vi "Append Changed Item.vi"(6 "change type":T1, 7 "item name":string, 9 "new value":string, 10 "old value":string, 11 "refresh items in":T2[](array[typedef])) -> (2 "modify parent":bool, 3 "refresh items out":T2[](array[typedef]))   [LabVIEW 2020, in "AIM MIL-STD-1553 System Explorer.lvlib" / "Implementation.lvlib" / "Refresh.lvlib"]
uses:
  Refresh.lvlib
  Change Type.ctl
  Symbols.ctl
  MCL Row.ctl
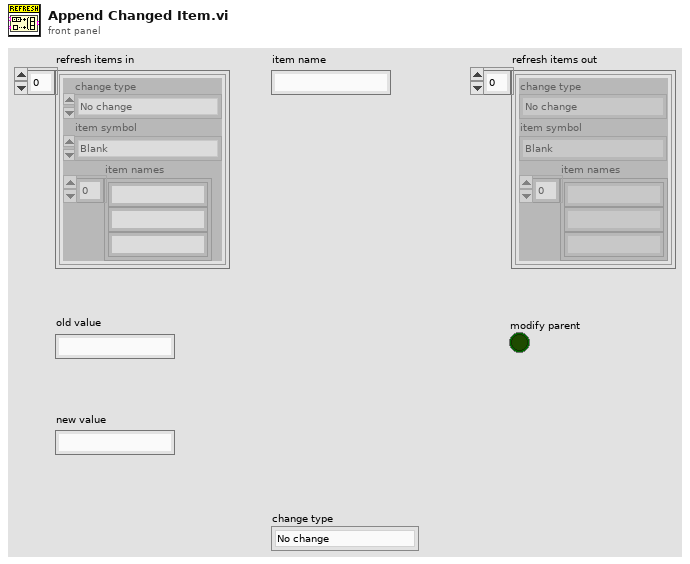
[diagram p1: front panel]
types:
  T1 = typedef "AIM MIL-STD-1553 System Explorer.lvlib/Implementation.lvlib/Refresh.lvlib/Change Type.ctl" = enum16{"No change", "Modify", "Add", "Remove"}
  T2 = typedef "AIM MIL-STD-1553 System Explorer.lvlib/Implementation.lvlib/Refresh.lvlib/MCL Row.ctl" = cluster{"change type":T1, "item symbol":T3, "item names":string[]}
  T3 = typedef "AIM MIL-STD-1553 System Explorer.lvlib/Implementation.lvlib/Refresh.lvlib/Symbols.ctl" = enum16{"Blank", "MIL-STD-1553", "Port", "Remote Terminal", "Subaddress", "Bus Controller", "Acyclic Frame", "Mode Code", "Message", "Parameter", "Item"}
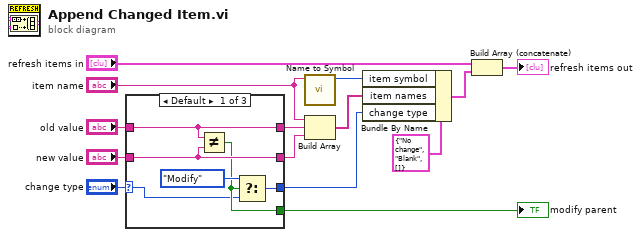
[diagram p0: block diagram]
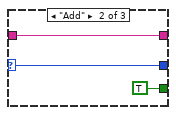
[diagram p2: hidden frame]
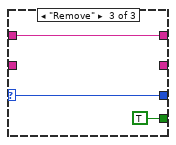
[diagram p3: hidden frame]
diagram:
  n1 = case shown="Default" "change type" {
    selector: "change type" -> [w15 w22 w25]
    tunnel: [w20 _ w26] -> w7
    tunnel: "old value" -> [w20 _ w26]
    tunnel: [w19 w23 _] -> w5
    tunnel: "new value" -> [w19 w23 _]
    tunnel: [w16 w22 w25] -> w2
    tunnel: [w17 TRUE TRUE] -> w1
    frame Default {
      n2 = Not Equal?(x=w20, y=w19) -> (x != y?=w17:bool)
      n3 = Select(t=Change_Type."Modify" ("y"), s=w17, f=w15) -> (s? t:f=w16:T1)
    }
    frame "Add" {
    }
    frame "Remove" {
    }
  }
  "modify parent" <- w1
  n4 = call "Name to Symbol.vi"("item name"="item name") -> ("item symbol"=w8:T3)  [unwired: 10 in]
  n5 = Build Array("item name", w7, w5) -> (w10:string[])
  n6 = Bundle By Name(cluster=T2 {"change type"=enum."No change", "item symbol"=enum."Blank", "item names"=[]} ("refresh listbox out"), "item symbol"=w8, "item names"=w10, "change type"=w2) -> (w12:T2)
  n7 = Build Array (concatenate)("refresh items in", w12) -> (→"refresh items out":T2[])
